vi "projetoIM_labview2021arduino.vi"() -> ()   [LabVIEW 2021]
uses:
  <vilib>/express/express arith-compare/Formula/XNode/ExpressFormulaBlockNode.xnode
  <vilib>/LabVIEW Interface for Arduino/LabVIEW Interface for Arduino.lvlib
panel:
  in  "Sample Rate":u16
  in  "Analog Pin":u8
  in  "Interface":enum16{"R5.00", "R6.25"}(ring)
  in  "Rg":enum16{"3k3", "1k5"}(ring)
  out "Força":dbl(knob) scale=0.0..10.0
  out "R_fsr":dbl
  out "Força":dbl
  out "Vout":dbl
  in  "stop":bool
  out "data":dynamicdata(graph) caption="Vout"
  # "mm"
  # "ohm"
  # "Arduino Controls"
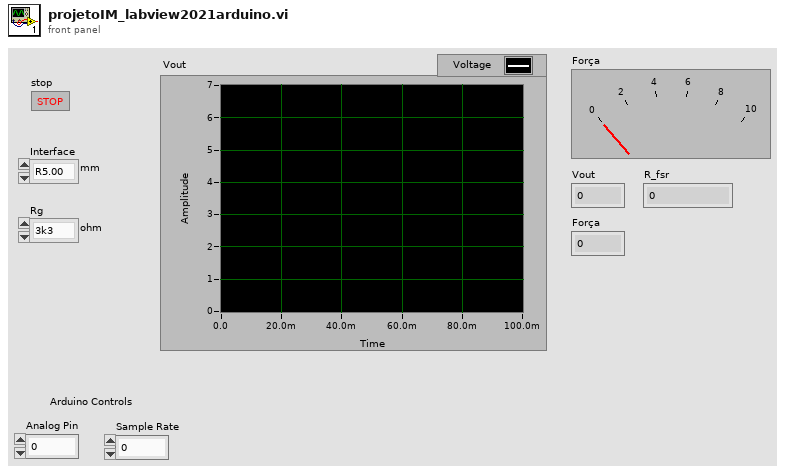
[diagram p1: front panel]
types:
  T1 = typedef "LabVIEW Interface for Arduino.lvlib/Arduino Resource.ctl" = cluster{"VISA resource":refnum<visa-resource-name>, "Board Type":T2, "Connection Type":enum8{"USB / Serial"}, "Bytes Per Packet (15)":u8}
  T2 = typedef "LabVIEW Interface for Arduino.lvlib/Board Type.ctl" = enum16{"Uno", "Dimuelanove w/Atmega 328", "Mega 2560"}
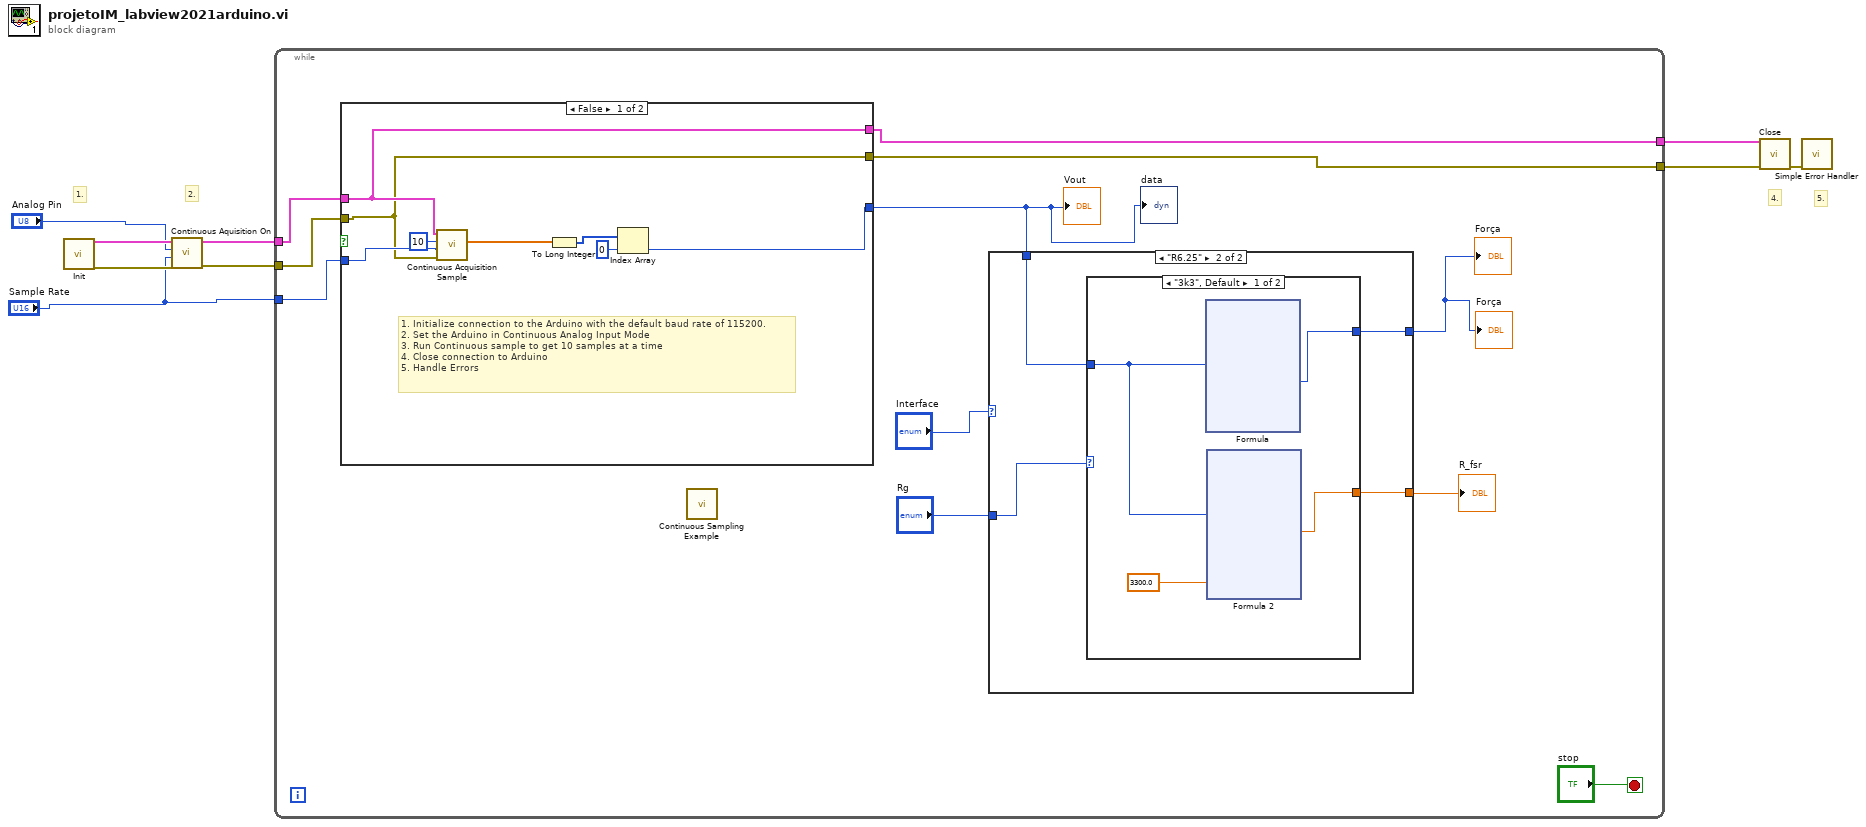
[diagram p0: block diagram]
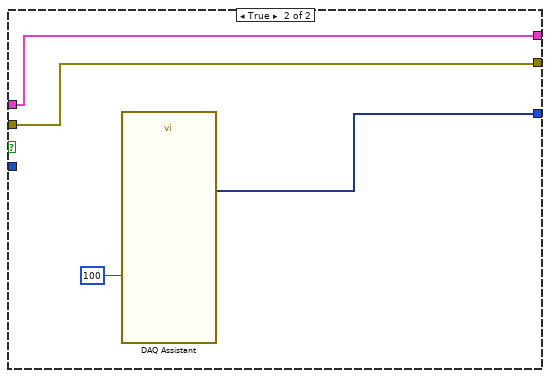
[diagram p2: hidden frame]
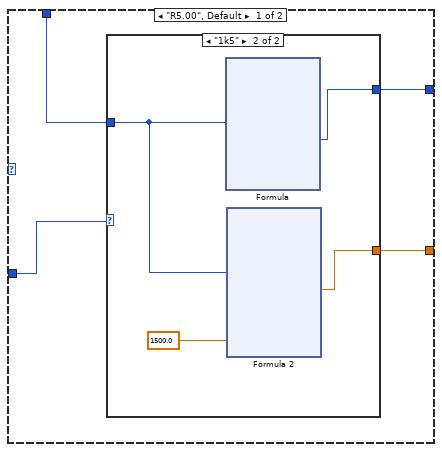
[diagram p3: hidden frame]
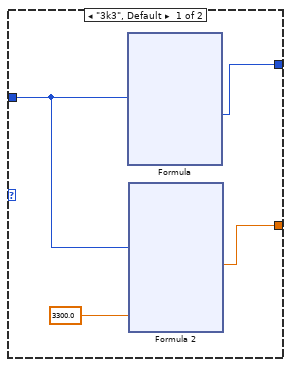
[diagram p4: hidden frame]
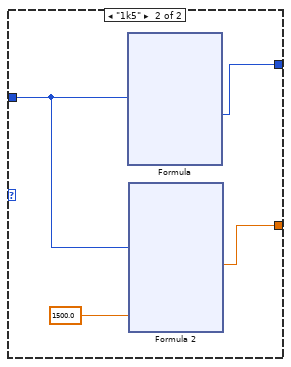
[diagram p5: hidden frame]
diagram:
  # "5."
  # "4."
  # "2."
  # "1."
  n1 = call <vilib>:"Init.vi"() -> ("Arduino Resource"=w7:T1, "error out"=w9:errorcluster)  [unwired: 18 in]
  n2 = call <vilib>:"Continuous Aquisition On.vi"("error in"=w9, "Acquition Speed"="Sample Rate", "Analog Input Pin"="Analog Pin", "Arduino Resource"=w7) -> ("error out"=w5:errorcluster, "Arduino Resource"=w6:T1)  [unwired: 6 in]
  n3 = while {
    tunnel: w6 -> [w13]
    tunnel: w5 -> [w14]
    tunnel: "Sample Rate" -> [w12]
    tunnel: [w11] -> w4
    tunnel: [w10] -> w3
    stop <- "stop" stop-if-true
    n4 = case shown="False" {
      selector: _ -> [_ _]
      tunnel: [w24 w31] -> w15
      tunnel: w14 -> [w21 w29]
      tunnel: w13 -> [w22 w30]
      tunnel: w12 -> [w27 _]
      tunnel: [w22 w30] -> w11
      tunnel: [w21 w29] -> w10
      frame False {
        # "1. Initialize connection to the Arduino with the default baud rate of 115200.\n2. Set the Arduino in Continuous Analog Input Mode\n3. Run Continuous sample to get 10 samples at a time\n4. Close connection to Arduino\n5. Handle Errors"
        n5 = call <vilib>:"Continuous Acquisition Sample.vi"("Arduino Resource"=w22, "Samples to Read"=u16 10, "Sample Rate (HZ)"=w27, "error in (no error)"=w21) -> ("Data"=w26:dbl[])  [unwired: 4 in, 2 out]
        n6 = To Long Integer(number=w26) -> (32bit integer=w25:i32[])
        n7 = Index Array(array=w25, index=0) -> (element=w24:i32)
      }
      frame True {
        n8 = call "DAQ Assistant"("number of samples"=100) -> ("data"=w31:dynamicdata)  [unwired: 16 in, 2 out]
      }
    }
    "data" <- w15
    "Vout" <- w15
    n9 = call <vilib>:"Continuous Sampling Example .vi"() -> ()  [unwired: 12 in]
    n10 = case shown="\"R6.25\"" "Interface" {
      tunnel: w15 -> [w36 w84]
      tunnel: [w35 w83] -> w18
      tunnel: [w34 w82] -> w19
      tunnel: "Rg" -> [w33 w81]
      frame "R5.00", Default {
        n11 = case shown="\"1k5\"" w33 {
          tunnel: w36 -> [w40 w62]
          tunnel: [w39 w61] -> w35
          tunnel: [w38 w60] -> w34
          frame "3k3", Default {
            n12 = xnode "Formula"("X1"=w40) -> ("Result"=w39:i32)  [unwired: 1 in, 1 out]
            n13 = xnode "Formula 2"("X1"=w40, "X2"=3300.0) -> ("Result"=w38:dbl)  [unwired: 1 in, 1 out]
          }
          frame "1k5" {
            n14 = xnode "Formula"("X1"=w62) -> ("Result"=w61:i32)  [unwired: 1 in, 1 out]
            n15 = xnode "Formula 2"("X1"=w62, "X2"=1500.0) -> ("Result"=w60:dbl)  [unwired: 1 in, 1 out]
          }
        }
      }
      frame "R6.25" {
        n16 = case shown="\"3k3\", Default" w81 {
          tunnel: w84 -> [w88 w110]
          tunnel: [w87 w109] -> w83
          tunnel: [w86 w108] -> w82
          frame "3k3", Default {
            n17 = xnode "Formula"("X1"=w88) -> ("Result"=w87:i32)  [unwired: 1 in, 1 out]
            n18 = xnode "Formula 2"("X1"=w88, "X2"=3300.0) -> ("Result"=w86:dbl)  [unwired: 1 in, 1 out]
          }
          frame "1k5" {
            n19 = xnode "Formula"("X1"=w110) -> ("Result"=w109:i32)  [unwired: 1 in, 1 out]
            n20 = xnode "Formula 2"("X1"=w110, "X2"=1500.0) -> ("Result"=w108:dbl)  [unwired: 1 in, 1 out]
          }
        }
      }
    }
    "Força" <- w18
    "R_fsr" <- w19
    "Força" <- w18
  }
  n21 = call <vilib>:"Close.vi"("Arduino Resource"=w4, "error in"=w3) -> ("error out"=w8:errorcluster)  [unwired: 13 in]
  n22 = call <vilib>:"Simple Error Handler.vi"("error in (no error)"=w8) -> ()  [unwired: 4 in, 5 out]
